vi "init server.vi"(8 "error in (no error)":errorcluster, 11 "Header content in":refnum<class "Header content.lvclass">) -> (0 "error out":errorcluster, 3 "Header content out":refnum<class "Header content.lvclass">)   [LabVIEW 2018, in "Header content.lvclass"]
uses:
  Header content.lvclass
  Server/Server.lvclass
  Server/Server.lvclass/Server.ctl
  Header content.lvclass/Header content.ctl
panel:
  in  "Server.lvclass":refnum<class "Server.lvclass">
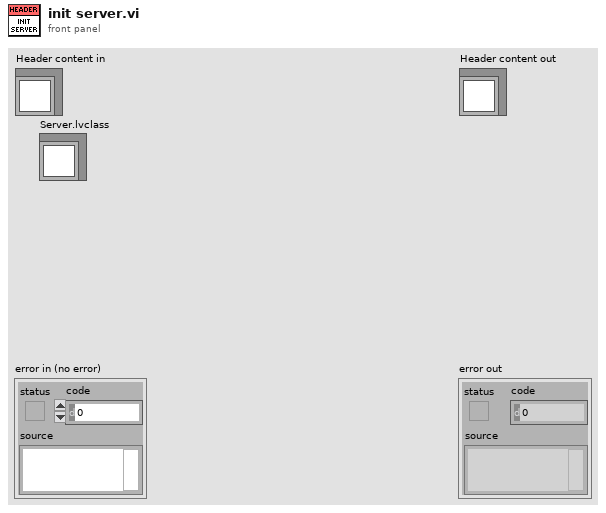
[diagram p1: front panel]
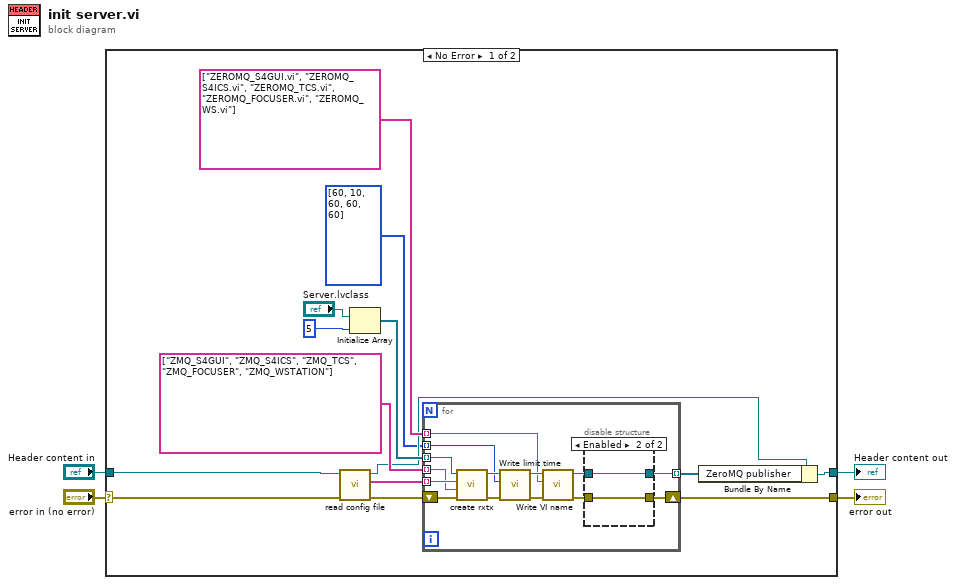
[diagram p0: block diagram]
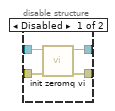
[diagram p2: hidden frame]
diagram:
  n1 = case shown="No Error" "error in (no error)" {
    selector: "error in (no error)" -> [w11 w40]
    tunnel: [w18 w40] -> w3
    tunnel: [w17 w39] -> w1
    tunnel: "Header content in" -> [w7 w39]
    frame No Error {
      n2 = call "read config file.vi"("error in (no error)"=w11, "Header content in"=w7) -> ("error out"=w10:errorcluster, "remote IPs"=w9:string[], "Header content out"=w6:refnum<class "Header content.lvclass">)  [unwired: 7 in]
      n3 = Initialize Array("Server.lvclass", 5 ("dimension size")) -> (w16:refnum<class "Server.lvclass">[])
      n4 = for {
        shift-right: [w21] -> w18
        shift-left: w10 -> [w32]
        tunnel: w9 -> [w28] mode=indexing
        tunnel: w16 -> [w30] mode=indexing
        tunnel: [w22] -> w14 mode=indexing
        tunnel: string[] ["ZMQ_S4GUI", "ZMQ_S4ICS", "ZMQ_TCS", "ZMQ_FOCUSER", "ZMQ_WSTATION"] -> [w27] mode=indexing
        tunnel: string[] ["ZEROMQ_S4GUI.vi", "ZEROMQ_S4ICS.vi", "ZEROMQ_TCS.vi", "ZEROMQ_FOCUSER.vi", "ZEROMQ_WS.vi"] -> [w20] mode=indexing
        tunnel: u16[] [60, 10, 60, 60, 60] -> [w19] mode=indexing
        n5 = call "create rxtx.vi"("error in (no error)"=w32, "qeue name"=w27, "remote IP"=w28, "Server in"=w30) -> ("error out"=w31:errorcluster, "Server out"=w29:refnum<class "Server.lvclass">)  [unwired: 6 in]
        n6 = call "Write limit time.vi"("error in (no error)"=w31, "limit time"=w19, "Server in"=w29) -> ("error out"=w24:errorcluster, "Server out"=w23:refnum<class "Server.lvclass">)  [unwired: 7 in]
        n7 = call "Write VI name.vi"("error in (no error)"=w24, "VI name"=w20, "Server in"=w23) -> ("error out"=w25:errorcluster, "Server out"=w26:refnum<class "Server.lvclass">)  [unwired: 7 in]
        n8 = disable-structure shown="Enabled" {
          disable-tunnel: w26 -> [w36 w38]
          disable-tunnel: w25 -> [w35 w37]
          disable-tunnel: [w34 w38] -> w22
          disable-tunnel: [w33 w37] -> w21
          frame Disabled {
            n9 = call "init zeromq vi.vi"("error in (no error)"=w35, "Server in"=w36) -> ("error out"=w33:errorcluster, "Server out"=w34:refnum<class "Server.lvclass">)  [unwired: 8 in]
          }
          frame Enabled {
          }
        }
      }
      n10 = Bundle By Name(cluster=w6, "ZeroMQ publisher"=w14) -> (w17:refnum<class "Header content.lvclass">)
    }
    frame Error {
    }
  }
  "error out" <- w3
  "Header content out" <- w1
